vi "Stimulus_timing_array_get.vi"(2 "minimum time between events":u32, 3 "experiment time":u32, 4 "array index":i32, 5 "timing array":dbl[](array[numeric])) -> (0 "index":i32, 1 "time":dbl)   [LabVIEW 2015]
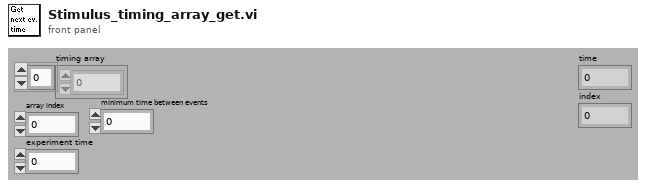
[diagram p1: front panel]
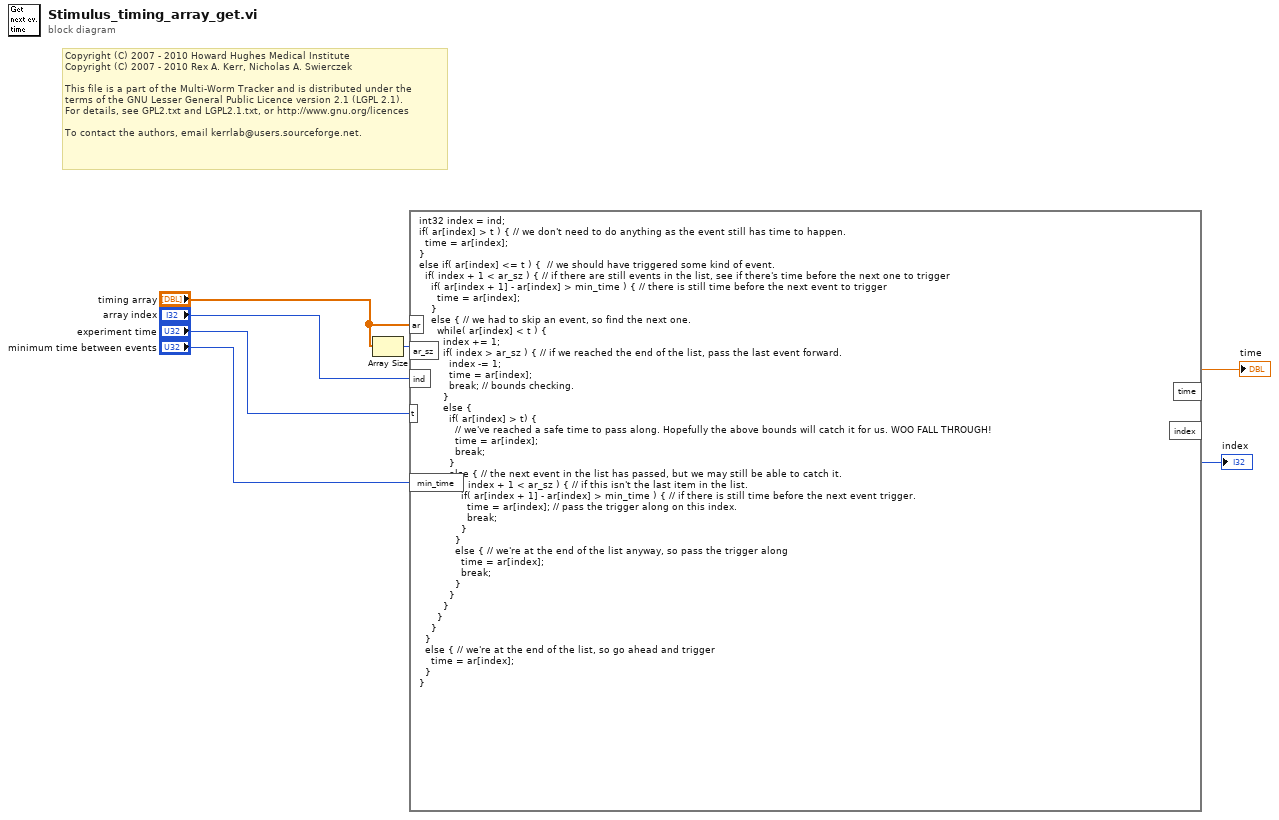
[diagram p0: block diagram]
diagram:
  # "Copyright (C) 2007 - 2010 Howard Hughes Medical Institute\nCopyright (C) 2007 - 2010 Rex A. Kerr, Nicholas A. Swierczek\n \nThis file is a part of the Multi-Worm Tracker and is distributed under the\nterms of the GNU Lesser General Public Licence version 2.1 (LGPL 2.1).\nFor details, see GPL2.txt and LGPL2.1.txt, or http://www.gnu.org/licences\n \nTo contact the authors, email kerrlab@users.sourceforge.net."
  n1 = Array Size(array="timing array") -> (size(s)=w3:i32)
  n2 = formula code="int32 index = ind;\nif( ar[index] > t ) { // we don't need to do anything as the event still has time to happen.\n  time = ar[index];\n}\nelse if( ar[index] <= t ) {  // we should have triggered some kind of event.\n  if( index + 1 < ar_sz ) { // if there are still events in the list, see if there's time before the next one to trigger\n    if( ar[index + 1] - ar[index] > min_time ) { // there is still time before the next event to trigger\n      time = ar[index];\n    }\n    else { // we had to skip an event, so find the next one.\n      while( ar[index] < t ) {\n        index += 1;\n        if( index > ar_sz ) { // if we reached the end of the list, pass the last event forward.\n          index -= 1;\n          time = ar[index];\n          break; // bounds checking.\n        }\n        else {\n          if( ar[index] > t) {\n            // we've reached a safe time to pass along. Hopefully the above bounds will catch it for us. WOO FALL THROUGH!\n            time = ar[index];\n            break;\n          }\n          else { // the next event in the list has passed, but we may still be able to catch it.\n            if( index + 1 < ar_sz ) { // if this isn't the last item in the list.\n              if( ar[index + 1] - ar[index] > min_time ) { // if there is still time before the next event trigger.\n                time = ar[index]; // pass the trigger along on this index.\n                break;\n              }\n            }\n            else { // we're at the end of the list anyway, so pass the trigger along\n              time = ar[index];\n              break;\n            }\n          }\n        }\n      }\n    }\n  }\n  else { // we're at the end of the list, so go ahead and trigger\n    time = ar[index];\n  }\n}"("ar"="timing array", "ind"="array index", "t"="experiment time", "min_time"="minimum time between events", "ar_sz"=w3) -> ("time"=→"time":dbl, "index"=→"index":i32)
